vi "ADC Get Current Setup.vi"(8 "error in":errorcluster, 11 "adc session in":T14={"niScope"={"channel cfg"=[], "sessions"=[], "multi cards"=FALSE, "channels"=0, "type"=enum."n/a", "memory [B/chn]"=0, "ext. clock [Hz]"=0.0, "samples count"=0, "use streaming"=FALSE, "proc setup"={"packet size [smpl]"=0, "current timeout [s]"=0.0, "blk2blk timeout [s]"=0.0, "event time"=timestamp(0 s since 1904-01-01), "temp sampl T [s]"=0.0, "data queue"=refnum, "stop notifier"=refnum, "proc ref"=refnum}, "sample width [B]"=0, "ranges [V]"=[], "trigger setup"={"coupling"=1, "level [V]"=0.0, "slope"=0, "mode"=enum."Immediate", "pre-trigger [%]"=0.0}, "fs [Hz]"=0.0, "bitres [bit]"=0, "clock source"=enum."VAL_NO_SOURCE"}, "3458A"={"channels"=[], "sync unit"={"VISA"="", "type"=enum."Picotest U6200A"}, "awg unit"={"type"=enum."Agilent 331xxA to 332xxA", "VISA"="", "enable 10MHz ref"=FALSE, "cmi ckd2"={"VISA"="", "clock source"=enum."Auto", "manual ref clk"=FALSE, "ref clock [Hz]"=0.0, "div mode"=enum."Set divisor directly"}, "cmi sync v3"={"VISA"="", "baud rate [bd/s]"=115200, "source"=enum."Auto", "hv range"=enum."1kV", "fsrc is fixed"=FALSE, "fsrc [Hz]"=10000000.0, "freq integ [s]"=1.0, "freq filter"=5, "trig level"=enum."TTL 5V", "chn1 mode"=enum."Source divider", "chn1 level"=enum."Positive 5V", "chn2 mode"=enum."Source divider", "chn2 level"=enum."Positive 5V", "chn2 div"=1, "chn3 mode"=enum."Chn 1 Active", "chn3 level"=enum."Positive 5V", "chn1 div entry"=enum."Calculate nearest divisor from measured fx", "chn1 dev limit [%]"=1.0, "chn1 check dev"=FALSE}, "trigger"={"source"=enum."Immediate", "slope"=enum."POS", "coupling"=enum."DC", "level [V]"=0.0, "hysteresis [V]"=0.0, "pre-trigger [%]"=0.0}, "HMF2500 cfg"={"Baud Rate"=9600, "Parity"=0, "Data Bits"=8, "Flow Control"=4}}, "sync mode"=enum."MASTER-SLAVE, MASTER clocked by TIMER", "streaming mode"=FALSE, "idn mode"=enum."Auto", "sampling mode"=enum."DCV", "sample memory [B]"=0, "proc setup"={"channel id"=0, "packet size [smpl]"=0, "current timeout [s]"=0.0, "blk2blk timeout [s]"=0.0, "event time"=timestamp(0 s since 1904-01-01), "stop notifier"=refnum, "data queues"=[], "proc refs"=[], "bus semaphore"=refnum}, "sample size [B]"=0, "sample count"=0, "aux data"={"channel id"=0, "valid?"=[], "gain [V]"=[], "timestamp [s]"=[], "Ts [s]"=0.0, "abs timestamp"=timestamp(0 s since 1904-01-01), "t [deg C]"=[], "multiplex timestamp [s]"=-1.0, "only multiplex?"=FALSE, "multiplex smpl offset"=0, "overflow?"=FALSE}, "ranges [V]"=[], "aperture [s]"=0.0, "LEVEL trigger"={"edge"=enum."POS", "level [V]"=0.0, "coupling"=enum."DC"}, "trigger mode"=enum."AUTO", "measure temp.?"=FALSE, "disp mesages"=[], "shared bus?"=FALSE, "disable display?"=FALSE, "aper mode"=enum."Manual", "aper rules"=[], "multiplex"={"cycles"=0, "delay [s]"=0.0, "enabled"=FALSE, "overhead [s]"=1.0, "tot smpls"=0, "sub-rec"=0, "overhead [%]"=0.0, "emulated"=FALSE}, "F8588 lpf"=enum."Off", "F8588 pll"=enum."Off", "F8588 couple"=enum."DC, auto", "fs"={"freq mode"=enum."fs or Ts", "fs [Hz]"=0.0, "fref [Hz]"=0.0, "mul"=0.0, "div"=0.0}, "fs mode"=enum."fs or Ts"}, "dsdll"={"dsdll"={"dsdll path"=path "", "dsdll handle"=[], "output devices"=[], "capture devices"=[]}, "channels"=0, "device id"=0, "channel idns"=[], "proc setup"={"packet size [smpl]"=0, "current timeout [s]"=0.0, "blk2blk timeout [s]"=0.0, "event time"=timestamp(0 s since 1904-01-01), "data queue"=refnum, "stop notifier"=refnum, "proc ref"=refnum}, "samples count"=0, "fs [Hz]"=0.0}, "type"=enum."niScope", "channel idn str"=[], "aux instr idn str"=[], "modified?"=FALSE, "simadc"={"channels"=[], "range [V]"=0.0, "Ts step [s]"=0.0, "time [s]"=0.0, "fs [Hz]"=0.0, "count"=0, "smpl offset"=0, "set count"=0, "bit res"=0}, "force rst?"=FALSE, "exit mode"=enum."Immediate reset", "exit dly"=0.0, "exit tmr"=timestamp(0 s since 1904-01-01), "busy?"=FALSE, "accessed?"=FALSE, "multiplex"={"Type"=enum."Dummy", "gen com ssn"={"visa"="", "primary"=enum."None", "secondary"=enum."None", "channels"=[]}, "delay before [s]"=0.0, "delay post [s]"=0.0, "sequence"=[], "enabled"=FALSE, "ref timestamp [s]"=0.0, "idn string"="", "dev niScope"="", "niScope idx"=0, "QPMX ssn"={"visa"="", "switch mode"=enum."Switched by TWM", "sequence"=[], "timing delays"=[], "polarity"=enum."Positive", "ss delay (s)"=2.0, "internal timer (s)"=1.0, "Last loaded sequence file"=path "", "startup delay (s)"=2.0}, "VISA mux ssn"={"VISA"="", "paths"=[], "idn command"="", "serial cfg"={"Baud rate"=9600, "Data bits"=8, "Parity"=0, "Stop bits"=10, "Flow control"=0, "End Mode Read"=enum."None", "End Mode Write"=enum."None", "Term character"=0, "Term enable"=FALSE}}}, "keysight dso"={"VISA"="", "channels"=[], "bw limit [Hz]"=0.0, "resolution"=enum."Basic", "trig noise reject"=enum."Normal", "N"=0, "trigger config"={"trigger source"=enum."Immediate", "trigger slope"=enum."Negative", "level [V]"=0.0, "hysteresis [V]"=0.001, "pre-trig [%]"=50}, "fs [Hz]"=0.0, "timeout stop"=timestamp(0 s since 1904-01-01), "waiting for opc"=FALSE, "fetch offset [smpl]"=0, "abs timestamp"=timestamp(0 s since 1904-01-01), "ranges [V]"=[], "decimation"=1.0, "ext ref"=FALSE, "emulate aperture"=FALSE, "model"=enum."DSO91304"}, "cdaq"={"mclk [Hz]"=12800000.0, "ADC task"="", "mclk reference"="", "fs [Hz]"=50000.0, "queue adc cmd"=refnum, "queue adc data"=refnum, "adc proc ref"=refnum, "channels"=[], "last channels"=[], "timeout"=timestamp(0 s since 1904-01-01), "N"=1000, "mclk mode"=enum."Free running", "ext mclk source"=""}, "ignore overload"=FALSE, "ADS127L21"={"VISA"="", "chn list"=[], "record size"=0, "phys. channels"=0, "adc fifo size"=0, "channels"=[], "ext refclk?"=FALSE, "fs [Hz]"=0.0, "ext refclk [Hz]"=0.0, "meas refclk [Hz]"=0.0, "EXTOUT mode"=enum."ADCCLK", "EXTOUT polarity"=enum."NORM", "EXTOUT divisor"=0}} {"ADS127L21"."channels"."Channel" min=1 max=8 step=1; "cdaq"."last channels"."Channel id" min=0 step=1; "cdaq"."channels"."Channel id" min=0 step=1; "keysight dso"."decimation" min=1.0; "keysight dso"."bw limit [Hz]" format="%#_6p"; "keysight dso"."channels"."Offset [V]" format="%#_6p"; "keysight dso"."channels"."Range [Vpk]" min=0.0 format="%#_6p"; "keysight dso"."channels"."Channel" min=1; "multiplex"."VISA mux ssn"."serial cfg"."Flow control" items=["None", "XON/XOFF", "CTS/RTS", "XON/XOFF + CTS/RTS", "DTR/DSR", "XON/XOFF + DTR/DSR"]; "multiplex"."VISA mux ssn"."serial cfg"."Stop bits" items=["1 bit"=10, "1.5 bits"=15, "2 bits"=20]; "multiplex"."VISA mux ssn"."serial cfg"."Parity" items=["None", "Odd", "Even", "Mark", "Space"]; "multiplex"."VISA mux ssn"."serial cfg"."Data bits" items=["5 bits"=5, "6 bits"=6, "7 bits"=7, "8 bits"=8]; "multiplex"."VISA mux ssn"."serial cfg"."Baud rate" items=["150 Bd"=150, "300 Bd"=300, "600 Bd"=600, "1200 Bd"=1200, "2400 Bd"=2400, "4800 Bd"=4800, "9600 Bd"=9600, "19.2 kBd"=19200, "38.4 kBd"=38400, "57.6 kBd"=57600, "115.2 kBd"=115200]; "multiplex"."QPMX ssn"."startup delay (s)" min=0.0 step=1.0; "multiplex"."QPMX ssn"."internal timer (s)" min=0.0 step=1.0; "multiplex"."QPMX ssn"."ss delay (s)" min=0.0 step=1.0; "multiplex"."QPMX ssn"."timing delays" min=1 max=255 step=1; "3458A"."awg unit"."HMF2500 cfg"."Flow Control" items=["None", "XON/XOFF", "RTS/CTS", "XON/XOFF & RTS/CTS", "DTR/DSR", "XON/XOFF & DTR/DSR"]; "3458A"."awg unit"."HMF2500 cfg"."Data Bits" items=["7"=7, "8"=8]; "3458A"."awg unit"."HMF2500 cfg"."Parity" items=["None", "Odd", "Even", "Mark", "Space"]; "3458A"."awg unit"."HMF2500 cfg"."Baud Rate" items=["300"=300, "600"=600, "1200"=1200, "2400"=2400, "4800"=4800, "9600"=9600, "19200"=19200]; "3458A"."awg unit"."cmi sync v3"."chn2 div" min=1 max=100000000 step=1; "3458A"."awg unit"."cmi sync v3"."fsrc [Hz]" format="%_8p"; "3458A"."channels"."Range [Vpk]" min=0.0; "niScope"."trigger setup"."pre-trigger [%]" format="%.2f"; "niScope"."trigger setup"."level [V]" format="%.2f"; "niScope"."trigger setup"."coupling" items=["AC"=0, "DC"=1, "HF Reject"=3, "LF Reject"=4, "AC Plus HF Reject"=1001]; "niScope"."channel cfg"."Range [Vpk]" min=0.0; "niScope"."channel cfg"."Channel" min=0}) -> (0 "error out":errorcluster, 1 "device specific attributes":T11[](array[typedef]), 2 "common attributes":T6, 3 "adc session out":T14={"niScope"={"channel cfg"=[], "sessions"=[], "multi cards"=FALSE, "channels"=0, "type"=enum."n/a", "memory [B/chn]"=0, "ext. clock [Hz]"=0.0, "samples count"=0, "use streaming"=FALSE, "proc setup"={"packet size [smpl]"=0, "current timeout [s]"=0.0, "blk2blk timeout [s]"=0.0, "event time"=timestamp(0 s since 1904-01-01), "temp sampl T [s]"=0.0, "data queue"=refnum, "stop notifier"=refnum, "proc ref"=refnum}, "sample width [B]"=0, "ranges [V]"=[], "trigger setup"={"coupling"=1, "level [V]"=0.0, "slope"=0, "mode"=enum."Immediate", "pre-trigger [%]"=0.0}, "fs [Hz]"=0.0, "bitres [bit]"=0, "clock source"=enum."VAL_NO_SOURCE"}, "3458A"={"channels"=[], "sync unit"={"VISA"="", "type"=enum."Picotest U6200A"}, "awg unit"={"type"=enum."Agilent 331xxA to 332xxA", "VISA"="", "enable 10MHz ref"=FALSE, "cmi ckd2"={"VISA"="", "clock source"=enum."Auto", "manual ref clk"=FALSE, "ref clock [Hz]"=0.0, "div mode"=enum."Set divisor directly"}, "cmi sync v3"={"VISA"="", "baud rate [bd/s]"=115200, "source"=enum."Auto", "hv range"=enum."1kV", "fsrc is fixed"=FALSE, "fsrc [Hz]"=10000000.0, "freq integ [s]"=1.0, "freq filter"=5, "trig level"=enum."TTL 5V", "chn1 mode"=enum."Source divider", "chn1 level"=enum."Positive 5V", "chn2 mode"=enum."Source divider", "chn2 level"=enum."Positive 5V", "chn2 div"=1, "chn3 mode"=enum."Chn 1 Active", "chn3 level"=enum."Positive 5V", "chn1 div entry"=enum."Calculate nearest divisor from measured fx", "chn1 dev limit [%]"=1.0, "chn1 check dev"=FALSE}, "trigger"={"source"=enum."Immediate", "slope"=enum."POS", "coupling"=enum."DC", "level [V]"=0.0, "hysteresis [V]"=0.0, "pre-trigger [%]"=0.0}, "HMF2500 cfg"={"Baud Rate"=9600, "Parity"=0, "Data Bits"=8, "Flow Control"=4}}, "sync mode"=enum."MASTER-SLAVE, MASTER clocked by TIMER", "streaming mode"=FALSE, "idn mode"=enum."Auto", "sampling mode"=enum."DCV", "sample memory [B]"=0, "proc setup"={"channel id"=0, "packet size [smpl]"=0, "current timeout [s]"=0.0, "blk2blk timeout [s]"=0.0, "event time"=timestamp(0 s since 1904-01-01), "stop notifier"=refnum, "data queues"=[], "proc refs"=[], "bus semaphore"=refnum}, "sample size [B]"=0, "sample count"=0, "aux data"={"channel id"=0, "valid?"=[], "gain [V]"=[], "timestamp [s]"=[], "Ts [s]"=0.0, "abs timestamp"=timestamp(0 s since 1904-01-01), "t [deg C]"=[], "multiplex timestamp [s]"=-1.0, "only multiplex?"=FALSE, "multiplex smpl offset"=0, "overflow?"=FALSE}, "ranges [V]"=[], "aperture [s]"=0.0, "LEVEL trigger"={"edge"=enum."POS", "level [V]"=0.0, "coupling"=enum."DC"}, "trigger mode"=enum."AUTO", "measure temp.?"=FALSE, "disp mesages"=[], "shared bus?"=FALSE, "disable display?"=FALSE, "aper mode"=enum."Manual", "aper rules"=[], "multiplex"={"cycles"=0, "delay [s]"=0.0, "enabled"=FALSE, "overhead [s]"=1.0, "tot smpls"=0, "sub-rec"=0, "overhead [%]"=0.0, "emulated"=FALSE}, "F8588 lpf"=enum."Off", "F8588 pll"=enum."Off", "F8588 couple"=enum."DC, auto", "fs"={"freq mode"=enum."fs or Ts", "fs [Hz]"=0.0, "fref [Hz]"=0.0, "mul"=0.0, "div"=0.0}, "fs mode"=enum."fs or Ts"}, "dsdll"={"dsdll"={"dsdll path"=path "", "dsdll handle"=[], "output devices"=[], "capture devices"=[]}, "channels"=0, "device id"=0, "channel idns"=[], "proc setup"={"packet size [smpl]"=0, "current timeout [s]"=0.0, "blk2blk timeout [s]"=0.0, "event time"=timestamp(0 s since 1904-01-01), "data queue"=refnum, "stop notifier"=refnum, "proc ref"=refnum}, "samples count"=0, "fs [Hz]"=0.0}, "type"=enum."niScope", "channel idn str"=[], "aux instr idn str"=[], "modified?"=FALSE, "simadc"={"channels"=[], "range [V]"=0.0, "Ts step [s]"=0.0, "time [s]"=0.0, "fs [Hz]"=0.0, "count"=0, "smpl offset"=0, "set count"=0, "bit res"=0}, "force rst?"=FALSE, "exit mode"=enum."Immediate reset", "exit dly"=0.0, "exit tmr"=timestamp(0 s since 1904-01-01), "busy?"=FALSE, "accessed?"=FALSE, "multiplex"={"Type"=enum."Dummy", "gen com ssn"={"visa"="", "primary"=enum."None", "secondary"=enum."None", "channels"=[]}, "delay before [s]"=0.0, "delay post [s]"=0.0, "sequence"=[], "enabled"=FALSE, "ref timestamp [s]"=0.0, "idn string"="", "dev niScope"="", "niScope idx"=0, "QPMX ssn"={"visa"="", "switch mode"=enum."Switched by TWM", "sequence"=[], "timing delays"=[], "polarity"=enum."Positive", "ss delay (s)"=2.0, "internal timer (s)"=1.0, "Last loaded sequence file"=path "", "startup delay (s)"=2.0}, "VISA mux ssn"={"VISA"="", "paths"=[], "idn command"="", "serial cfg"={"Baud rate"=9600, "Data bits"=8, "Parity"=0, "Stop bits"=10, "Flow control"=0, "End Mode Read"=enum."None", "End Mode Write"=enum."None", "Term character"=0, "Term enable"=FALSE}}}, "keysight dso"={"VISA"="", "channels"=[], "bw limit [Hz]"=0.0, "resolution"=enum."Basic", "trig noise reject"=enum."Normal", "N"=0, "trigger config"={"trigger source"=enum."Immediate", "trigger slope"=enum."Negative", "level [V]"=0.0, "hysteresis [V]"=0.001, "pre-trig [%]"=50}, "fs [Hz]"=0.0, "timeout stop"=timestamp(0 s since 1904-01-01), "waiting for opc"=FALSE, "fetch offset [smpl]"=0, "abs timestamp"=timestamp(0 s since 1904-01-01), "ranges [V]"=[], "decimation"=1.0, "ext ref"=FALSE, "emulate aperture"=FALSE, "model"=enum."DSO91304"}, "cdaq"={"mclk [Hz]"=12800000.0, "ADC task"="", "mclk reference"="", "fs [Hz]"=50000.0, "queue adc cmd"=refnum, "queue adc data"=refnum, "adc proc ref"=refnum, "channels"=[], "last channels"=[], "timeout"=timestamp(0 s since 1904-01-01), "N"=1000, "mclk mode"=enum."Free running", "ext mclk source"=""}, "ignore overload"=FALSE, "ADS127L21"={"VISA"="", "chn list"=[], "record size"=0, "phys. channels"=0, "adc fifo size"=0, "channels"=[], "ext refclk?"=FALSE, "fs [Hz]"=0.0, "ext refclk [Hz]"=0.0, "meas refclk [Hz]"=0.0, "EXTOUT mode"=enum."ADCCLK", "EXTOUT polarity"=enum."NORM", "EXTOUT divisor"=0}} {"ADS127L21"."channels"."Channel" min=1 max=8 step=1; "cdaq"."last channels"."Channel id" min=0 step=1; "cdaq"."channels"."Channel id" min=0 step=1; "keysight dso"."decimation" min=1.0; "keysight dso"."bw limit [Hz]" format="%#_6p"; "keysight dso"."channels"."Offset [V]" format="%#_6p"; "keysight dso"."channels"."Range [Vpk]" min=0.0 format="%#_6p"; "keysight dso"."channels"."Channel" min=1; "multiplex"."VISA mux ssn"."serial cfg"."Flow control" items=["None", "XON/XOFF", "CTS/RTS", "XON/XOFF + CTS/RTS", "DTR/DSR", "XON/XOFF + DTR/DSR"]; "multiplex"."VISA mux ssn"."serial cfg"."Stop bits" items=["1 bit"=10, "1.5 bits"=15, "2 bits"=20]; "multiplex"."VISA mux ssn"."serial cfg"."Parity" items=["None", "Odd", "Even", "Mark", "Space"]; "multiplex"."VISA mux ssn"."serial cfg"."Data bits" items=["5 bits"=5, "6 bits"=6, "7 bits"=7, "8 bits"=8]; "multiplex"."VISA mux ssn"."serial cfg"."Baud rate" items=["150 Bd"=150, "300 Bd"=300, "600 Bd"=600, "1200 Bd"=1200, "2400 Bd"=2400, "4800 Bd"=4800, "9600 Bd"=9600, "19.2 kBd"=19200, "38.4 kBd"=38400, "57.6 kBd"=57600, "115.2 kBd"=115200]; "multiplex"."QPMX ssn"."startup delay (s)" min=0.0 step=1.0; "multiplex"."QPMX ssn"."internal timer (s)" min=0.0 step=1.0; "multiplex"."QPMX ssn"."ss delay (s)" min=0.0 step=1.0; "multiplex"."QPMX ssn"."timing delays" min=1 max=255 step=1; "3458A"."awg unit"."HMF2500 cfg"."Flow Control" items=["None", "XON/XOFF", "RTS/CTS", "XON/XOFF & RTS/CTS", "DTR/DSR", "XON/XOFF & DTR/DSR"]; "3458A"."awg unit"."HMF2500 cfg"."Data Bits" items=["7"=7, "8"=8]; "3458A"."awg unit"."HMF2500 cfg"."Parity" items=["None", "Odd", "Even", "Mark", "Space"]; "3458A"."awg unit"."HMF2500 cfg"."Baud Rate" items=["300"=300, "600"=600, "1200"=1200, "2400"=2400, "4800"=4800, "9600"=9600, "19200"=19200]; "3458A"."awg unit"."cmi sync v3"."chn2 div" min=1 max=100000000 step=1; "3458A"."awg unit"."cmi sync v3"."fsrc [Hz]" format="%_8p"; "3458A"."channels"."Range [Vpk]" min=0.0; "niScope"."trigger setup"."pre-trigger [%]" format="%.2f"; "niScope"."trigger setup"."level [V]" format="%.2f"; "niScope"."trigger setup"."coupling" items=["AC"=0, "DC"=1, "HF Reject"=3, "LF Reject"=4, "AC Plus HF Reject"=1001]; "niScope"."channel cfg"."Range [Vpk]" min=0.0; "niScope"."channel cfg"."Channel" min=0})   [LabVIEW 2020]
doc: "Returns current setup of the ADC (from session) so it will correctly work only after 'ADC Setup Virtual Channels'. It also returns device specific attributes as and array of names and text values."
uses:
  ADC Session.ctl
  drivers/niScope/niScope Session.ctl
  drivers/niScope/niScope Virtual Channel Config.ctl
  drivers/niScope/niScope Virtual Channel Mode.ctl
  drivers/niScope/niScope Virtual Channel Input Z.ctl
  drivers/niScope/niScope Virtual Channel Coupling.ctl
  drivers/niScope/niScope Type.ctl
  drivers/niScope/niScope Digitizing Process Options.ctl
  drivers/niScope/niScope Data Packet.ctl
  drivers/niScope/niScope Trigger Setup.ctl
  <instrlib>/niScope/Controls/niScope trigger coupling.ctl
  <instrlib>/niScope/Controls/niScope trigger slope.ctl
  drivers/niScope/niScope Reference Clock.ctl
  drivers/DMM/3458A Digitizer Session.ctl
  drivers/DMM/3458A Virtual Channel Config.ctl
  drivers/Counter/Counter Session.ctl
  drivers/Counter/Counter Type.ctl
  drivers/AWG/AWG Session.ctl
  drivers/AWG/AWG Type.ctl
  drivers/AWG/CMI Clock Divider v2/CMI ckd2 Session.ctl
  drivers/AWG/CMI Clock Divider v2/CMI ckd2 Source Mode.ctl
  drivers/AWG/CMI Clock Divider v2/CMI ckd2 Divisor Mode.ctl
  drivers/AWG/CMI Sync V3/CMI Sync V3 session.ctl
  drivers/AWG/CMI Sync V3/Configure/CMI Sync V3 Reference Clock Source.ctl
  drivers/AWG/CMI Sync V3/Configure/CMI Sync V3 HV input Range.ctl
  drivers/AWG/CMI Sync V3/Configure/CMI Sync V3 Trigger Input Level.ctl
  drivers/AWG/CMI Sync V3/Configure/CMI Sync V3 Channel 1 Mode.ctl
  drivers/AWG/CMI Sync V3/Configure/CMI Sync V3 Channel Output Levels.ctl
  drivers/AWG/CMI Sync V3/Configure/CMI Sync V3 Channel 2 Mode.ctl
  drivers/AWG/CMI Sync V3/Configure/CMI Sync V3 Channel 3 Mode.ctl
  drivers/AWG/CMI Sync V3/Configure/CMI Sync V3 Channel 1 Divisor Entry Mode.ctl
  ADC Trig Config.ctl
  ADC Trig Mode Source.ctl
  ADC Trig Slope.ctl
  ADC Trig Coupling.ctl
  drivers/AWG/RaS HMF2500/HMF2500 Config.ctl
  drivers/DMM/3458A Sync Mode.ctl
  drivers/DMM/3458A Idn Mode.ctl
  drivers/DMM/3458A Digitizing Low Levels/Configure/Sampling Mode.ctl
  drivers/DMM/3458A Digitizing Process Options.ctl
  drivers/DMM/3458A Data Packet.ctl
  drivers/DMM/3458A Aux Record Data.ctl
  drivers/DMM/3458A Digitizing Low Levels/Configure/Level Setup.ctl
  drivers/DMM/3458A Digitizing Low Levels/Configure/First Sample Trigger.ctl
  drivers/DMM/3458A Aperture Selection Mode.ctl
  drivers/DMM/3458A Multiplexing Config.ctl
  drivers/Fluke 8588A/F8588A Low Pass Filter.ctl
  drivers/Fluke 8588A/F8588A Phase Lock.ctl
  drivers/Fluke 8588A/F8588A Coupling.ctl
  drivers/DMM/3458A Sampling Rate.ctl
  drivers/AWG/AWG Clock Setup Mode.ctl
  drivers/DMM/3458A Sample Rate Mode.ctl
  drivers/dsdll/DSDLL Session.ctl
  drivers/dsdll/dsdll/dsdll_instance.ctl
  drivers/dsdll/dsdll/dsdll_device_record.ctl
  drivers/dsdll/DSDLL Process Config.ctl
  drivers/dsdll/DSDLL Data Packet.ctl
  ADC Type.ctl
  drivers/simulated_adc/SimAdc Config.ctl
  drivers/simulated_adc/SimAdc Channel Cfg.ctl
  ADC On Close Action.ctl
  Multiplexer/MPX Session.ctl
  Multiplexer/MPX Type.ctl
  drivers/Multiplexers/Generic COM/GCOMM Session.ctl
  drivers/Multiplexers/Generic COM/GCOMM Signal.ctl
  drivers/Multiplexers/Generic COM/GCOMM Virtual Channel.ctl
  drivers/Multiplexers/Generic COM/GCOMM Logic State.ctl
  drivers/Multiplexers/Generic COM/QPMX Session.ctl
  drivers/Multiplexers/QPMX/QPMX switch mode.ctl
  drivers/Multiplexers/QPMX/QPMX polarity.ctl
  drivers/Multiplexers/Generic VISA commands/GVISA Mux Session.ctl
  drivers/Multiplexers/Generic VISA commands/GVISA Mux Path Entry.ctl
  drivers/Multiplexers/Generic VISA commands/met_serial_setup.ctl
  drivers/Agilent DSO 90000/Virtual Digitizer/KeDSO session.ctl
  drivers/Agilent DSO 90000/Virtual Digitizer/KeDSO Virtual Channel.ctl
  drivers/Agilent DSO 90000/Virtual Digitizer/KeDSO High Resolution Mode.ctl
  drivers/Agilent DSO 90000/Virtual Digitizer/KeDSO Trigger Setup.ctl
  drivers/Agilent DSO 90000/Virtual Digitizer/KeDSO Trigger Source.ctl
  drivers/Agilent DSO 90000/Public/Utility/DSO type.ctl
  drivers/cdaq/cDAQ Session.ctl
  drivers/cdaq/low_level_old/cdaq_anal_adc_command.ctl
  drivers/cdaq/low_level_old/cdaq_anal_adc_data.ctl
  drivers/cdaq/cDAQ Virtual Channel.ctl
  drivers/cdaq/cDAQ Master Clock Mode.ctl
  drivers/CMI_ADS127L21/CMI ADS127L21 - Session.ctl
  drivers/CMI_ADS127L21/CMI ADS127L21 - Record Channel.ctl
  drivers/CMI_ADS127L21/CMI ADS127L21 - Input Range.ctl
  drivers/CMI_ADS127L21/CMI ADS127L21 - Input Mode.ctl
  drivers/CMI_ADS127L21/CMI ADS127L21 - Input Impedance.ctl
  drivers/CMI_ADS127L21/CMI ADS127L21 - EXTOUT Mode.ctl
  drivers/CMI_ADS127L21/CMI ADS127L21 - EXTOUT Polarity.ctl
  ADC Attribute.ctl
  ADC Current Configuration.ctl
  drivers/DMM/3458A Virtual Digitizer.lvlib
  drivers/niScope/niScope Virtual Digitizer.lvlib
  drivers/Counter/Counter.lvlib
  drivers/AWG/AWG.lvlib
  drivers/DMM/3458A Digitizing Low Levels/3458A Digitizing Low Levels.lvlib
  drivers/dsdll/DSDLL Virtual Digitizer.lvlib
  drivers/dsdll/dsdll/dsdll.lvlib
  drivers/AWG/CMI Sync V3/CMI Sync Unit V3.lvlib
  drivers/Agilent DSO 90000/Agilent 90000 Series.lvlib
panel:
  in  "ads127 Impedance":T1
  in  "ads127 Mode":T2
  in  "Coupling 2":enum16{"DC", "DC50", "AC", "LFR1"}(ring)
  in  "Coupling":T3=enum."DC"
  in  "Input Z":T4
  in  "Mode":T5
  in  "3458A.sync mode":T12
  in  "3458A.sampling mode":T13
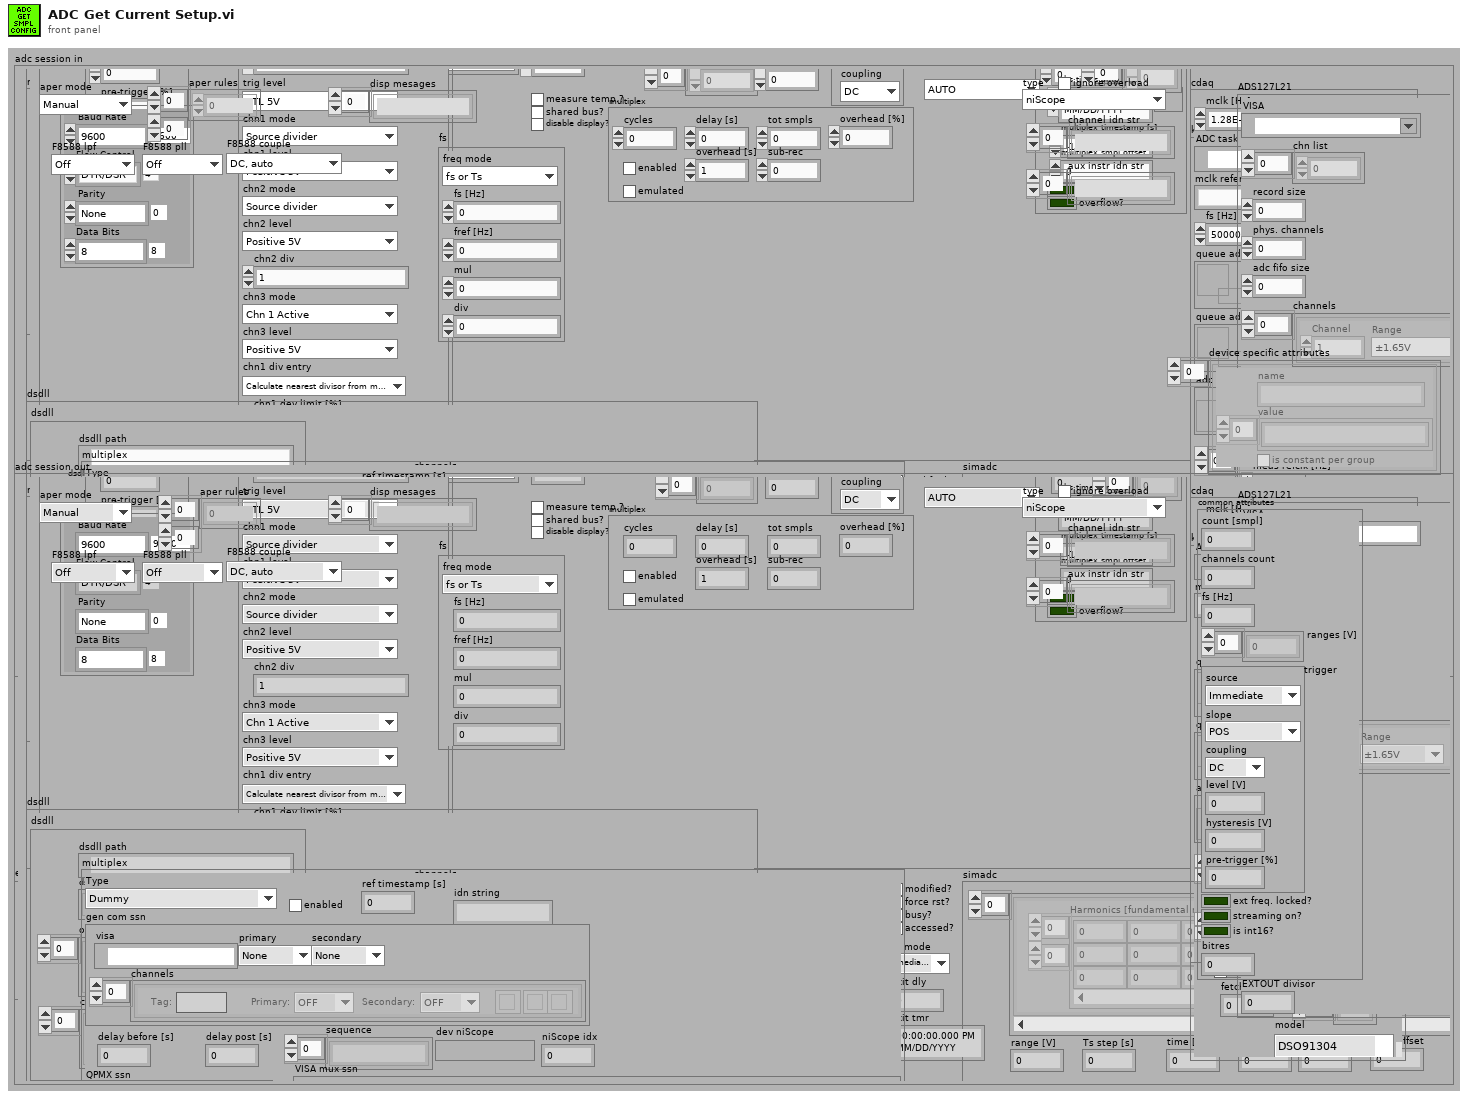
[diagram p1: front panel]
types:
  T1 = typedef "CMI ADS127L21 - Input Impedance.ctl" = enum16{"1M", "1k5"}
  T2 = typedef "CMI ADS127L21 - Input Mode.ctl" = enum16{"Normal", "Inverted", "GND"}
  T3 = typedef "niScope Virtual Digitizer.lvlib/niScope Virtual Channel Coupling.ctl" = enum16{"AC", "DC", "GND"}
  T4 = typedef "niScope Virtual Digitizer.lvlib/niScope Virtual Channel Input Z.ctl" = enum16{"1 MOhm", "50 Ohm"}
  T5 = typedef "niScope Virtual Digitizer.lvlib/niScope Virtual Channel Mode.ctl" = enum16{"Single ended", "Unbal. differential", "Differential"}
  T6 = typedef "ADC Current Configuration.ctl" = cluster{"count [smpl]":i64, "channels count":i32, "fs [Hz]":dbl, "ranges [V]":dbl[], "trigger":T7, "ext freq. locked?":bool, "streaming on?":bool, "is int16?":bool, "bitres":i32}
  T7 = typedef "ADC Trig Config.ctl" = cluster{"source":T8, "slope":T9, "coupling":T10, "level [V]":dbl, "hysteresis [V]":dbl, "pre-trigger [%]":dbl}
  T8 = typedef "ADC Trig Mode Source.ctl" = enum16{"Immediate", "External", "Level"}
  T9 = typedef "ADC Trig Slope.ctl" = enum16{"POS", "NEG"}
  T10 = typedef "ADC Trig Coupling.ctl" = enum16{"DC", "AC"}
  T11 = typedef "ADC Attribute.ctl" = cluster{"name":string, "value":string[], "is constant per group":bool}
  T12 = typedef "3458A Virtual Digitizer.lvlib/3458A Sync Mode.ctl" = enum16{"MASTER-SLAVE, MASTER clocked by TIMER", "MASTER-SLAVE, MASTER clocked by AWG", "ALL clocked by AWG", "MASTER-SLAVE, ALL clocked by TIMER", "ALL clocked by AWG with DFLL"}
  T13 = typedef "3458A Virtual Digitizer.lvlib/3458A Digitizing Low Levels.lvlib/Sampling Mode.ctl" = enum16{"DCV", "DSDC", "DSAC"}
  T14 = typedef "ADC Session.ctl" = cluster{"niScope":T15, "3458A":T23, "dsdll":T56, "type":T60, "channel idn str":string[], "aux instr idn str":string[], "modified?":bool, "simadc":T61, "force rst?":bool, "exit mode":T63, "exit dly":dbl, "exit tmr":timestamp, "busy?":bool, "accessed?":bool, "multiplex":T64, "keysight dso":T76, "cdaq":T82, "ignore overload":bool, "ADS127L21":T85}
  T15 = typedef "niScope Virtual Digitizer.lvlib/niScope Session.ctl" = cluster{"channel cfg":T16[], "sessions":refnum<k20>[], "multi cards":bool, "channels":i32, "type":T17, "memory [B/chn]":i32, "ext. clock [Hz]":dbl, "samples count":i64, "use streaming":bool, "proc setup":T18, "sample width [B]":i32, "ranges [V]":dbl[], "trigger setup":T19, "fs [Hz]":dbl, "bitres [bit]":i32, "clock source":T22}
  T16 = typedef "niScope Virtual Digitizer.lvlib/niScope Virtual Channel Config.ctl" = cluster{"Address":refnum<k15>, "Channel":i32, "Mode":T5, "Input Z":T4, "Coupling":T3, "Range [Vpk]":dbl, "btn clr":bool, "btn up":bool, "btn down":bool}
  T17 = typedef "niScope Virtual Digitizer.lvlib/niScope Type.ctl" = enum16{"n/a", "5922"}
  T18 = typedef "niScope Virtual Digitizer.lvlib/niScope Digitizing Process Options.ctl" = cluster{"packet size [smpl]":i64, "current timeout [s]":dbl, "blk2blk timeout [s]":dbl, "event time":timestamp, "temp sampl T [s]":dbl, "data queue":refnum<queue>, "stop notifier":refnum<notifier>, "proc ref":refnum<vi>}
  T19 = typedef "niScope Virtual Digitizer.lvlib/niScope Trigger Setup.ctl" = cluster{"coupling":T20, "level [V]":dbl, "slope":T21, "mode":enum16{"Immediate", "External", "Level"}, "pre-trigger [%]":dbl}
  T20 = typedef "niScope trigger coupling.ctl" = u16
  T21 = typedef "niScope trigger slope.ctl" = i32
  T22 = typedef "niScope Virtual Digitizer.lvlib/niScope Reference Clock.ctl" = enum16{"VAL_NO_SOURCE", "VAL_CLK_IN", "VAL_PXI_CLOCK", "VAL_EXTERNAL"}
  T23 = typedef "3458A Virtual Digitizer.lvlib/3458A Digitizer Session.ctl" = cluster{"channels":T24[], "sync unit":T25, "awg unit":T27, "sync mode":T12, "streaming mode":bool, "idn mode":T42, "sampling mode":T13, "sample memory [B]":i32, "proc setup":T43, "sample size [B]":i32, "sample count":i32, "aux data":T45, "ranges [V]":dbl[], "aperture [s]":dbl, "LEVEL trigger":T46, "trigger mode":T47, "measure temp.?":bool, "disp mesages":string[], "shared bus?":bool, "disable display?":bool, "aper mode":T48, "aper rules":dbl[][], "multiplex":T49, "F8588 lpf":T50, "F8588 pll":T51, "F8588 couple":T52, "fs":T53, "fs mode":T55}
  T24 = typedef "3458A Virtual Digitizer.lvlib/3458A Virtual Channel Config.ctl" = cluster{"VISA":refnum<visa-resource-name>, "Range [Vpk]":dbl, "btn clr":bool, "btn up":bool, "btn down":bool, "F8588":bool, "F8588 guard":bool}
  T25 = typedef "Counter.lvlib/Counter Session.ctl" = cluster{"VISA":refnum<visa-resource-name>, "type":T26}
  T26 = typedef "Counter.lvlib/Counter Type.ctl" = enum16{"Picotest U6200A", "dummy"}
  T27 = typedef "AWG.lvlib/AWG Session.ctl" = cluster{"type":T28, "VISA":refnum<visa-resource-name>, "enable 10MHz ref":bool, "cmi ckd2":T29, "cmi sync v3":T32, "trigger":T7, "HMF2500 cfg":T41}
  T28 = typedef "AWG.lvlib/AWG Type.ctl" = enum16{"Agilent 331xxA to 332xxA", "Agilent 335xxA to 336xxA", "Tektronix AFG3101C", "R&S HMF25xx", "CMI Clock Divider v2", "CMI Sync Unit V3", "dummy"}
  T29 = typedef "AWG.lvlib/CMI ckd2 Session.ctl" = cluster{"VISA":refnum<visa-resource-name>, "clock source":T30, "manual ref clk":bool, "ref clock [Hz]":dbl, "div mode":T31}
  T30 = typedef "AWG.lvlib/CMI ckd2 Source Mode.ctl" = enum16{"Auto", "LF clock", "HF clock", "Internal"}
  T31 = typedef "AWG.lvlib/CMI ckd2 Divisor Mode.ctl" = enum16{"Set divisor directly", "Set divisor by frequency"}
  T32 = typedef "AWG.lvlib/CMI Sync Unit V3.lvlib/CMI Sync V3 session.ctl" = cluster{"VISA":refnum<visa-resource-name>, "baud rate [bd/s]":i32, "source":T33, "hv range":T34, "fsrc is fixed":bool, "fsrc [Hz]":dbl, "freq integ [s]":dbl, "freq filter":i32, "trig level":T35, "chn1 mode":T36, "chn1 level":T37, "chn2 mode":T38, "chn2 level":T37, "chn2 div":i32, "chn3 mode":T39, "chn3 level":T37, "chn1 div entry":T40, "chn1 dev limit [%]":dbl, "chn1 check dev":bool}
  T33 = typedef "AWG.lvlib/CMI Sync Unit V3.lvlib/CMI Sync V3 Reference Clock Source.ctl" = enum16{"Auto", "Internal", "Logic", "Sine", "HV"}
  T34 = typedef "AWG.lvlib/CMI Sync Unit V3.lvlib/CMI Sync V3 HV input Range.ctl" = enum16{"10V", "60V", "250V", "1kV"}
  T35 = typedef "AWG.lvlib/CMI Sync Unit V3.lvlib/CMI Sync V3 Trigger Input Level.ctl" = enum16{"LVCMOS 3V3", "TTL 5V"}
  T36 = typedef "AWG.lvlib/CMI Sync Unit V3.lvlib/CMI Sync V3 Channel 1 Mode.ctl" = enum16{"Source divider", "DDS absolute", "DDS ratio", "DDS ratio M/N"}
  T37 = typedef "AWG.lvlib/CMI Sync Unit V3.lvlib/CMI Sync V3 Channel Output Levels.ctl" = enum16{"Positive 3V3", "Negative 3V3", "Positive 5V", "Negative 5V"}
  T38 = typedef "AWG.lvlib/CMI Sync Unit V3.lvlib/CMI Sync V3 Channel 2 Mode.ctl" = enum16{"Source divider", "Chn 1 divide"}
  T39 = typedef "AWG.lvlib/CMI Sync Unit V3.lvlib/CMI Sync V3 Channel 3 Mode.ctl" = enum16{"Chn 1 Active", "Chn 2 Active", "Chn 1 Trigger", "Chn 2 Trigger", "Gate", "PPS", "10MHz"}
  T40 = typedef "AWG.lvlib/CMI Sync Unit V3.lvlib/CMI Sync V3 Channel 1 Divisor Entry Mode.ctl" = enum16{"Set divisor directly", "Calculate nearest divisor from measured fx"}
  T41 = typedef "AWG.lvlib/HMF2500 Config.ctl" = cluster{"Baud Rate":u32, "Parity":u16, "Data Bits":u16, "Flow Control":u16}
  T42 = typedef "3458A Virtual Digitizer.lvlib/3458A Idn Mode.ctl" = enum16{"Auto", "Sequential (chn A, chn B, ...)", "From calibration string"}
  T43 = typedef "3458A Virtual Digitizer.lvlib/3458A Digitizing Process Options.ctl" = cluster{"channel id":i32, "packet size [smpl]":i32, "current timeout [s]":dbl, "blk2blk timeout [s]":dbl, "event time":timestamp, "stop notifier":refnum<notifier>, "data queues":refnum<queue>[], "proc refs":refnum<vi>[], "bus semaphore":T44}
  T44 = typedef "Semaphore RefNum" = refnum<k1>
  T45 = typedef "3458A Virtual Digitizer.lvlib/3458A Aux Record Data.ctl" = cluster{"channel id":i32, "valid?":bool[], "gain [V]":dbl[], "timestamp [s]":dbl[], "Ts [s]":dbl, "abs timestamp":timestamp, "t [deg C]":dbl[], "multiplex timestamp [s]":dbl, "only multiplex?":bool, "multiplex smpl offset":i64, "overflow?":bool}
  T46 = typedef "3458A Virtual Digitizer.lvlib/3458A Digitizing Low Levels.lvlib/Level Setup.ctl" = cluster{"edge":enum16{"POS", "NEG"}, "level [V]":dbl, "coupling":enum16{"DC", "AC"}}
  T47 = typedef "3458A Virtual Digitizer.lvlib/3458A Digitizing Low Levels.lvlib/First Sample Trigger.ctl" = enum16{"AUTO", "EXT", "SYN", "SGL", "HOLD", "LEVEL"}
  T48 = typedef "3458A Virtual Digitizer.lvlib/3458A Aperture Selection Mode.ctl" = enum16{"Manual", "Maximum", "Table"}
  T49 = typedef "3458A Virtual Digitizer.lvlib/3458A Multiplexing Config.ctl" = cluster{"cycles":i32, "delay [s]":dbl, "enabled":bool, "overhead [s]":dbl, "tot smpls":i64, "sub-rec":i32, "overhead [%]":dbl, "emulated":bool}
  T50 = typedef "F8588A Low Pass Filter.ctl" = enum16{"Off", "100 kHz", "3 MHz"}
  T51 = typedef "F8588A Phase Lock.ctl" = enum16{"Off", "1 MHz", "10 MHz"}
  T52 = typedef "F8588A Coupling.ctl" = enum16{"AC, 1 MOhm", "AC, 10 MOhm", "DC, 1 MOhm", "DC, 10 MOhm", "DC, auto"}
  T53 = typedef "3458A Virtual Digitizer.lvlib/3458A Sampling Rate.ctl" = cluster{"freq mode":T54, "fs [Hz]":dbl, "fref [Hz]":dbl, "mul":dbl, "div":dbl}
  T54 = typedef "AWG.lvlib/AWG Clock Setup Mode.ctl" = enum16{"fs or Ts", "fs or Ts with fref", "fref/N", "fref*M/N", "fref*Ratio"}
  T55 = typedef "3458A Sample Rate Mode.ctl" = enum16{"fs or Ts", "fs*M/N"}
  T56 = typedef "DSDLL Virtual Digitizer.lvlib/DSDLL Session.ctl" = cluster{"dsdll":T57, "channels":i32, "device id":i32, "channel idns":string[], "proc setup":T59, "samples count":i32, "fs [Hz]":dbl}
  T57 = typedef "dsdll.lvlib/dsdll_instance.ctl" = cluster{"dsdll path":path, "dsdll handle":u8[], "output devices":T58[], "capture devices":T58[]}
  T58 = typedef "dsdll.lvlib/dsdll_device_record.ctl" = cluster{"guid":u8[], "name":string}
  T59 = typedef "DSDLL Virtual Digitizer.lvlib/DSDLL Process Config.ctl" = cluster{"packet size [smpl]":i32, "current timeout [s]":dbl, "blk2blk timeout [s]":dbl, "event time":timestamp, "data queue":refnum<queue>, "stop notifier":refnum<notifier>, "proc ref":refnum<vi>}
  T60 = typedef "ADC Type.ctl" = enum16{"niScope", "3458A", "DirectSound DLL", "Keysight DSO", "cDAQ ADC", "CMI ADS127L21", "dummy"}
  T61 = typedef "SimAdc Config.ctl" = cluster{"channels":T62[], "range [V]":dbl, "Ts step [s]":dbl, "time [s]":dbl, "fs [Hz]":dbl, "count":i64, "smpl offset":i64, "set count":i64, "bit res":i32}
  T62 = typedef "SimAdc Channel Cfg.ctl" = cluster{"harmonics":dbl[][], "btn clear":bool, "noise":dbl, "fundamental [Hz]":dbl}
  T63 = typedef "ADC On Close Action.ctl" = enum16{"Immediate reset", "Delayed reset"}
  T64 = typedef "MPX Session.ctl" = cluster{"Type":T65, "gen com ssn":T66, "delay before [s]":dbl, "delay post [s]":dbl, "sequence":string[], "enabled":bool, "ref timestamp [s]":dbl, "idn string":string, "dev niScope":refnum<k15>, "niScope idx":i32, "QPMX ssn":T70, "VISA mux ssn":T73}
  T65 = typedef "MPX Type.ctl" = enum16{"Dummy", "Generic - COM port", "Generic - niScope PFI", "Generic - VISA commands", "QPMX"}
  T66 = typedef "GCOMM Session.ctl" = cluster{"visa":refnum<visa-resource-name>, "primary":T67, "secondary":T67, "channels":T68[]}
  T67 = typedef "GCOMM Signal.ctl" = enum16{"None", "DTR", "RTS"}
  T68 = typedef "GCOMM Virtual Channel.ctl" = cluster{"Primary:":T69, "Secondary:":T69, "btn clr":bool, "btn up":bool, "btn down":bool, "Tag:":string}
  T69 = typedef "GCOMM Logic State.ctl" = enum16{"OFF", "ON"}
  T70 = typedef "QPMX Session.ctl" = cluster{"visa":refnum<visa-resource-name>, "switch mode":T71, "sequence":bool[][], "timing delays":u32[], "polarity":T72, "ss delay (s)":dbl, "internal timer (s)":dbl, "Last loaded sequence file":path, "startup delay (s)":dbl}
  T71 = typedef "QPMX switch mode.ctl" = enum16{"Switched by TWM", "Switched by external clock", "Switched by internal clock"}
  T72 = typedef "QPMX polarity.ctl" = enum16{"Positive", "Negative"}
  T73 = typedef "GVISA Mux Session.ctl" = cluster{"VISA":refnum<visa-resource-name>, "paths":T74[], "idn command":string, "serial cfg":T75}
  T74 = typedef "GVISA Mux Path Entry.ctl" = cluster{"Tag:":string, "Command:":string, "btn clr":bool, "btn up":bool, "btn down":bool}
  T75 = typedef "met_serial_setup.ctl" = cluster{"Baud rate":i32, "Data bits":i32, "Parity":i32, "Stop bits":i32, "Flow control":i32, "End Mode Read":enum16{"None", "Last Bit", "TermChar"}, "End Mode Write":enum16{"None", "Last Bit", "TermChar"}, "Term character":u8, "Term enable":bool}
  T76 = typedef "KeDSO session.ctl" = cluster{"VISA":refnum<visa-resource-name>, "channels":T77[], "bw limit [Hz]":dbl, "resolution":T78, "trig noise reject":enum16{"Normal", "High Sensitivity"}, "N":i64, "trigger config":T79, "fs [Hz]":dbl, "timeout stop":timestamp, "waiting for opc":bool, "fetch offset [smpl]":i64, "abs timestamp":timestamp, "ranges [V]":dbl[], "decimation":dbl, "ext ref":bool, "emulate aperture":bool, "model":T81}
  T77 = typedef "KeDSO Virtual Channel.ctl" = cluster{"Channel":i32, "Range [Vpk]":dbl, "btn clr":bool, "btn up":bool, "btn down":bool, "Offset [V]":dbl, "Coupling":enum16{"DC", "DC50", "AC", "LFR1"}, "bw limit enab":bool}
  T78 = typedef "KeDSO High Resolution Mode.ctl" = enum16{"Basic", "High-res AUTO", "Min. 9-bits", "Min. 10-bits", "Min. 11-bits", "Min. 12-bits", "Fixed 11-bits", "Fixed 12-bits", "Fixed 13-bits", "Fixed 14-bits", "Fixed 15-bits", "Fixed 16-bits"}
  T79 = typedef "KeDSO Trigger Setup.ctl" = cluster{"trigger source":T80, "trigger slope":enum16{"Negative", "Positive", "Either"}, "level [V]":dbl, "hysteresis [V]":dbl, "pre-trig [%]":i32}
  T80 = typedef "KeDSO Trigger Source.ctl" = enum16{"Immediate", "Level", "AUX"}
  T81 = typedef "Agilent 90000 Series.lvlib/DSO type.ctl" = enum16{"DSO91304", "DSO91204", "DSO90804", "DSO90604", "DSO90404", "DSO90254", "DSA91304", "DSA91204", "DSA90804", "DSA90604", "DSA90404", "DSA90254", "DSO9104", "DSO9254", "DSO9404", "MSO9104", "MSO9254", "MSO9404", "MSO9064", "DSO9064", "DSOX91604", "DSOX92004", "DSOX92504", "DSOX92804", "DSOX93204", "DSO93004", "DSO9024H", "DSO9054H", "DSO9104H", "DSO9204H", "DSOS054A", "DSOS104A", "DSOS204A", "DSOS254A", "DSOS404A", "DSOS604A", "DSOS804A", "MSOS054A", "MSOS104A", "MSOS204A", "MSOS254A", "MSOS404A", "MSOS604A", "MSOS804A", "DSAX96204Q", "DSOX96204Q", "DSAX95004Q", "DSOX95004Q", "DSAX93304Q", "DSOX93304Q", "DSAX92504Q", "DSOX92504Q", "DSAX92004Q", "DSOX92004Q"}
  T82 = typedef "cDAQ Session.ctl" = cluster{"mclk [Hz]":dbl, "ADC task":refnum<k21>, "mclk reference":string, "fs [Hz]":dbl, "queue adc cmd":refnum<queue>, "queue adc data":refnum<queue>, "adc proc ref":refnum<vi>, "channels":T83[], "last channels":T83[], "timeout":timestamp, "N":i32, "mclk mode":T84, "ext mclk source":tag}
  T83 = typedef "cDAQ Virtual Channel.ctl" = cluster{"Device":tag, "Channel id":i32, "btn clr":bool, "btn up":bool, "btn down":bool}
  T84 = typedef "cDAQ Master Clock Mode.ctl" = enum16{"Free running", "Export master clock", "Import master clock"}
  T85 = typedef "CMI ADS127L21 - Session.ctl" = cluster{"VISA":refnum<visa-resource-name>, "chn list":i32[], "record size":i32, "phys. channels":i32, "adc fifo size":i32, "channels":T86[], "ext refclk?":bool, "fs [Hz]":dbl, "ext refclk [Hz]":dbl, "meas refclk [Hz]":dbl, "EXTOUT mode":T88, "EXTOUT polarity":T89, "EXTOUT divisor":i32}
  T86 = typedef "CMI ADS127L21 - Record Channel.ctl" = cluster{"Range":T87, "Channel":i32, "Mode":T2, "Impedance":T1}
  T87 = typedef "CMI ADS127L21 - Input Range.ctl" = enum16{"±1.65V", "±2V"}
  T88 = typedef "CMI ADS127L21 - EXTOUT Mode.ctl" = enum16{"ADCCLK", "REFCLK", "SMPLCLK", "FIRST"}
  T89 = typedef "CMI ADS127L21 - EXTOUT Polarity.ctl" = enum16{"NORM", "INV"}
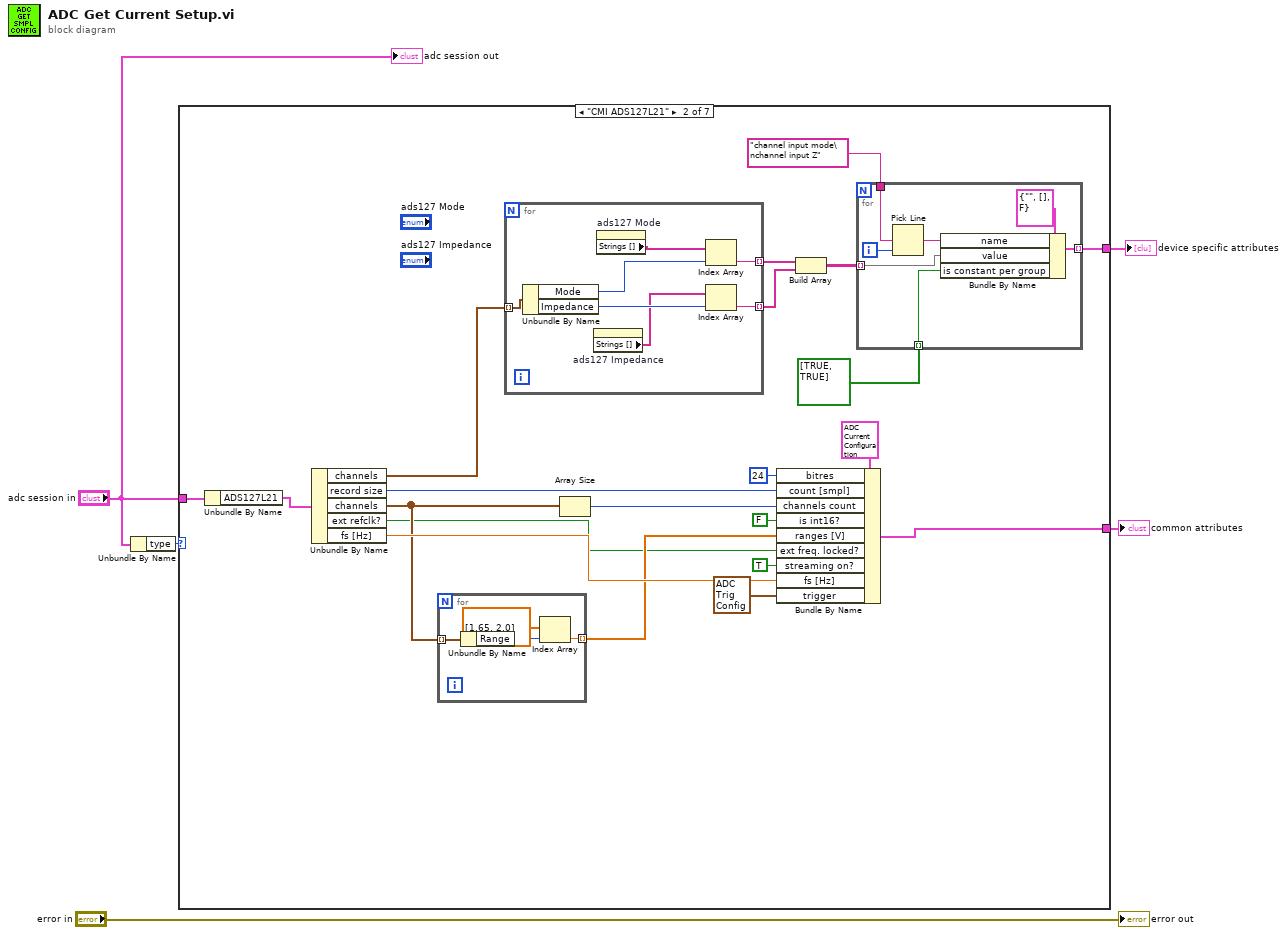
[diagram p0: block diagram]
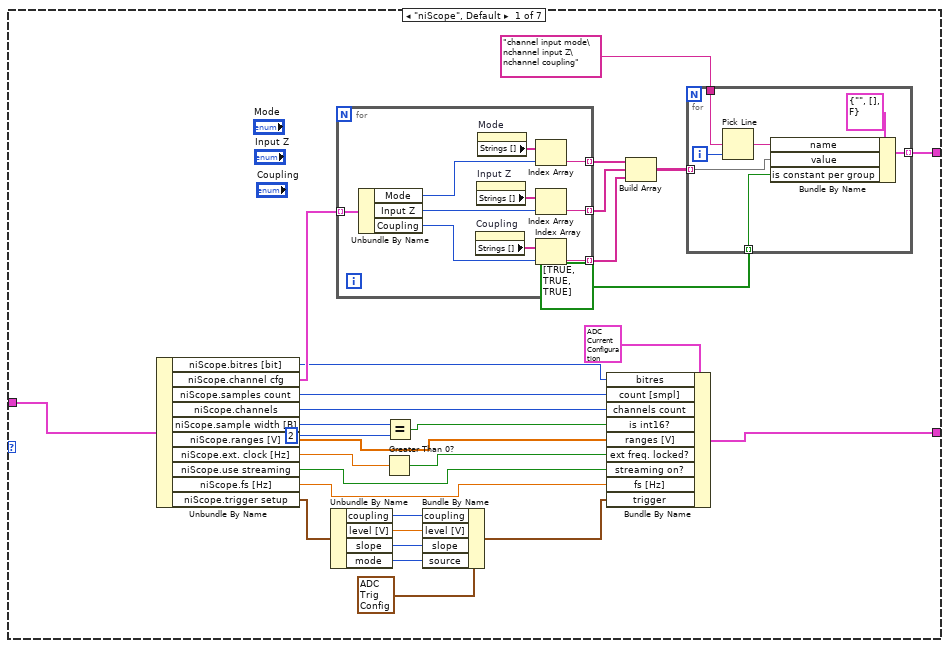
[diagram p2: hidden frame]
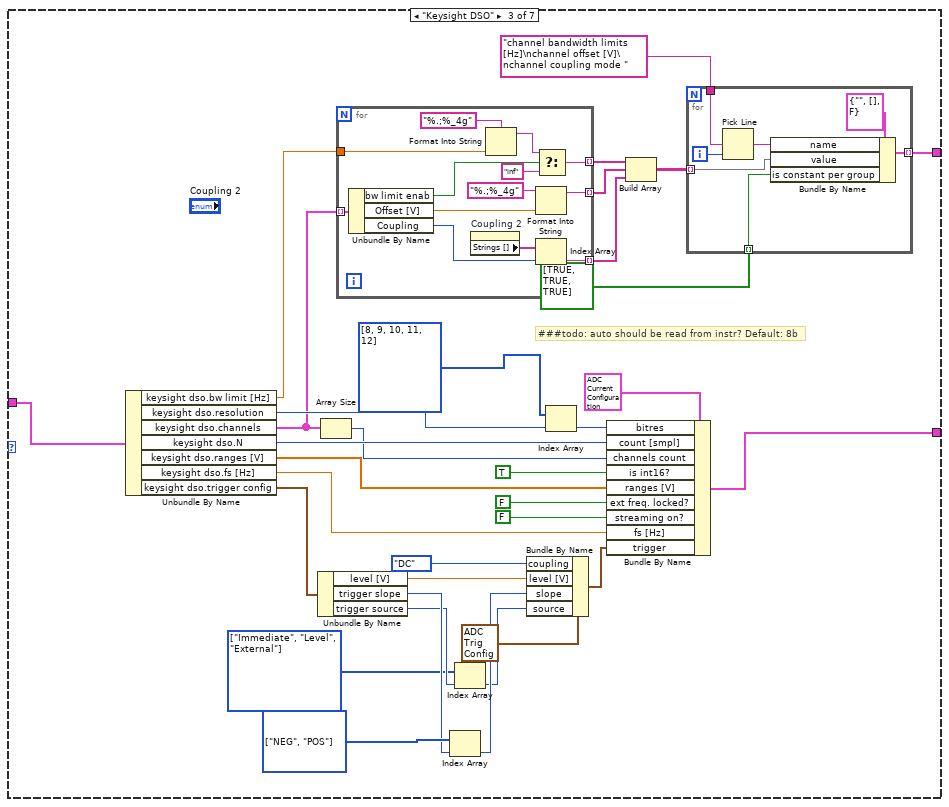
[diagram p3: hidden frame]
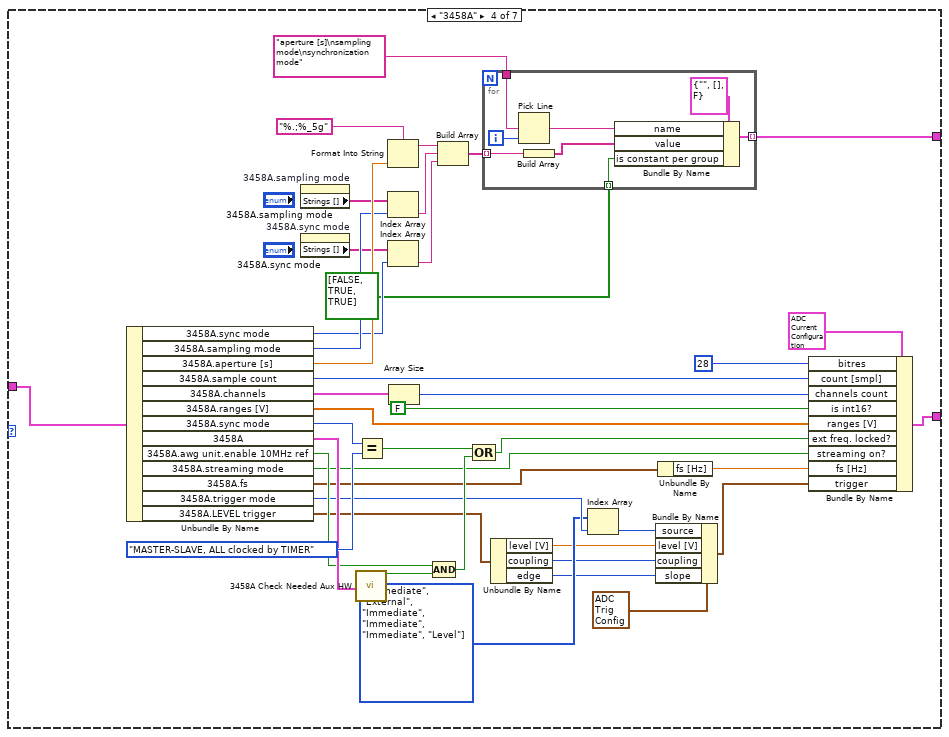
[diagram p4: hidden frame]
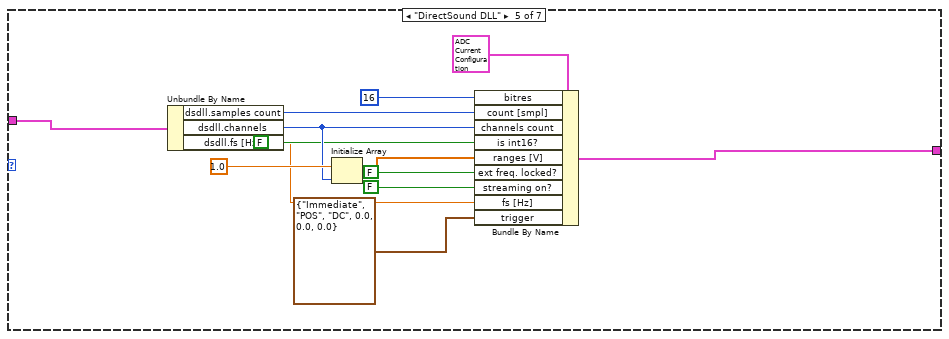
[diagram p5: hidden frame]
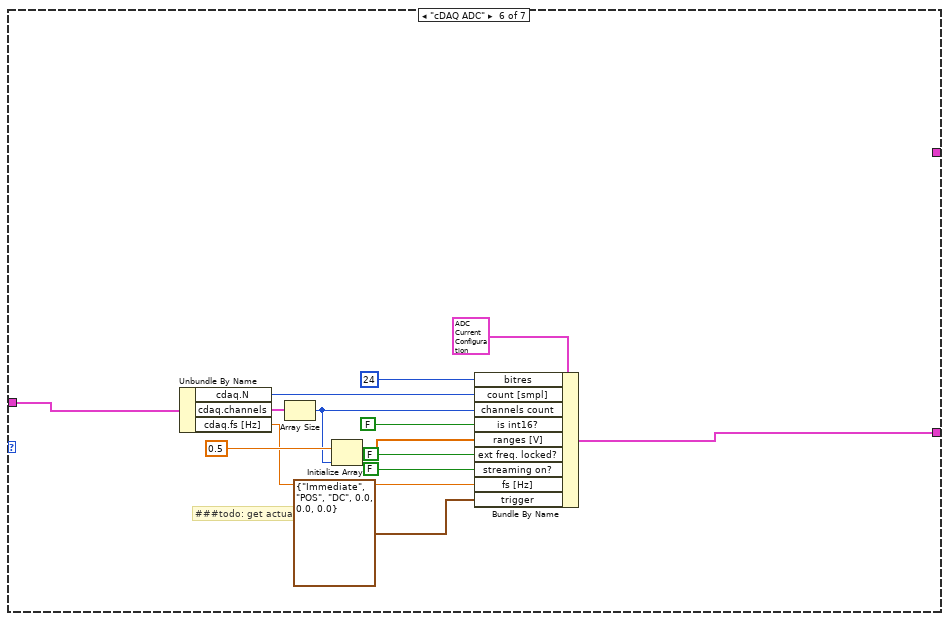
[diagram p6: hidden frame]
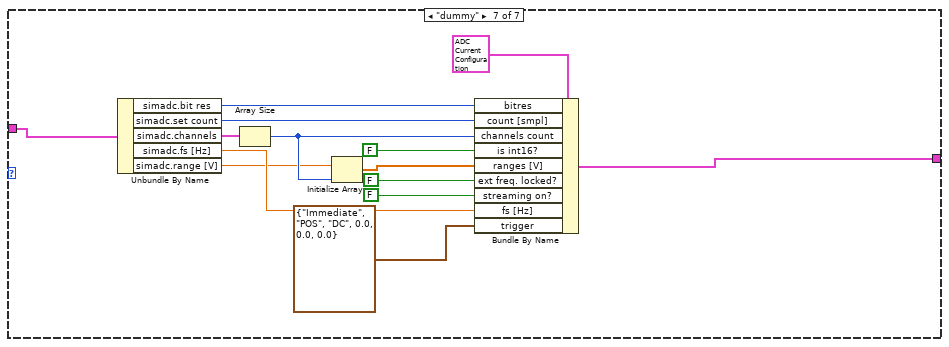
[diagram p7: hidden frame]
diagram:
  n1 = Unbundle By Name("adc session in") -> ("type"=w5:T60)
  n2 = case shown="\"CMI ADS127L21\"" w5 {
    tunnel: "adc session in" -> [w34 w61 w123 w185 w206 w220 w234]
    tunnel: [w8 w63 w108 w172 _ _ _] -> w2
    tunnel: [w23 w70 w119 w158 w197 w211 w227] -> w1
    frame "niScope", Default {
      n3 = Unbundle By Name(w34) -> ("niScope.bitres [bit]"=w7:i32, "niScope.channel cfg"=w14:T16[], "niScope.samples count"=w30:i64, "niScope.channels"=w29:i32, "niScope.sample width [B]"=w33:i32, "niScope.ranges [V]"=w27:dbl[], "niScope.ext. clock [Hz]"=w26:dbl, "niScope.use streaming"=w24:bool, "niScope.fs [Hz]"=w22:dbl, "niScope.trigger setup"=w21:T19)
      n4 = Unbundle By Name(w21) -> ("coupling"=w19:T20, "level [V]"=w18:dbl, "slope"=w17:T21, "mode"=w16:enum16{"Immediate", "External", "Level"})
      n5 = for {
        tunnel: w14 -> [w51] mode=indexing
        tunnel: [w48] -> w12 mode=indexing
        tunnel: [w45] -> w11 mode=indexing
        tunnel: [w42] -> w10 mode=indexing
        n6 = Unbundle By Name(w51) -> ("Mode"=w50:T5, "Input Z"=w46:T4, "Coupling"=w43:T3)
        n7 = property on="Coupling" class="Enum (strict)"() -> ("Strings []"=w44:string[])  [unwired: 2 in, 2 out]
        n8 = property on="Input Z" class="Enum (strict)"() -> ("Strings []"=w47:string[])  [unwired: 2 in, 2 out]
        n9 = property on="Mode" class="Enum (strict)"() -> ("Strings []"=w49:string[])  [unwired: 2 in, 2 out]
        n10 = Index Array(array=w49, index=w50) -> (element=w48:string)
        n11 = Index Array(array=w47, index=w46) -> (element=w45:string)
        n12 = Index Array(array=w44, index=w43) -> (element=w42:string)
      }
      n13 = Greater Than 0?(x=w26) -> (x > 0?=w25:bool)
      n14 = Equal?(x=w33, y=2) -> (x = y?=w28:bool)
      n15 = Bundle By Name(cluster=T7 {"source"=enum."Immediate", "slope"=enum."POS", "coupling"=enum."DC", "level [V]"=0.0, "hysteresis [V]"=0.0, "pre-trigger [%]"=0.0} ("trigger"), "coupling"=w19, "level [V]"=w18, "slope"=w17, "source"=w16) -> (w15:T7)
      n16 = Bundle By Name(cluster=T6 {"count [smpl]"=0, "channels count"=0, "fs [Hz]"=0.0, "ranges [V]"=[], "trigger"={"source"=enum."Immediate", "slope"=enum."POS", "coupling"=enum."DC", "level [V]"=0.0, "hysteresis [V]"=0.0, "pre-trigger [%]"=0.0}, "ext freq. locked?"=FALSE, "streaming on?"=FALSE, "is int16?"=FALSE, "bitres"=0} ("common attributes"), "bitres"=w7, "count [smpl]"=w30, "channels count"=w29, "is int16?"=w28, "ranges [V]"=w27, "ext freq. locked?"=w25, "streaming on?"=w24, "fs [Hz]"=w22, "trigger"=w15) -> (w23:T6)
      n17 = Build Array(w12, w11, w10) -> (w9:string[][])
      n18 = for {
        tunnel: "channel input mode\nchannel input Z\nchannel coupling" -> [w40]
        tunnel: [w37] -> w8 mode=indexing
        tunnel: w9 -> [w36] mode=indexing
        tunnel: bool[] [TRUE, TRUE, TRUE] -> [w35] mode=indexing
        i -> [w39]
        n19 = Pick Line(multi-line string=w40, line index=w39) -> (output string=w38:string)  [unwired: 1 in]
        n20 = Bundle By Name(cluster=T11 {"name"="", "value"=[], "is constant per group"=FALSE} ("adc attribute"), "name"=w38, "value"=w36, "is constant per group"=w35) -> (w37:T11)
      }
    }
    frame "CMI ADS127L21" {
      n21 = Unbundle By Name(w61) -> ("ADS127L21"=w60:T85)
      n22 = Unbundle By Name(w60) -> ("channels"=w68:T86[], "record size"=w71:i32, "channels"=w56:T86[], "ext refclk?"=w54:bool, "fs [Hz]"=w69:dbl)
      n23 = for {
        tunnel: w56 -> [w76] mode=indexing
        tunnel: [w73] -> w55 mode=indexing
        n24 = Unbundle By Name(w76) -> ("Range"=w75:T87)
        n25 = Index Array(array=dbl[] [1.65, 2.0], index=w75) -> (element=w73:dbl)
      }
      n26 = for {
        tunnel: w68 -> [w90] mode=indexing
        tunnel: [w88] -> w66 mode=indexing
        tunnel: [w86] -> w65 mode=indexing
        n27 = Unbundle By Name(w90) -> ("Mode"=w89:T2, "Impedance"=w87:T1)
        n28 = property on="ads127 Impedance" class="Enum (strict)"() -> ("Strings []"=w84:string[])  [unwired: 2 in, 2 out]
        n29 = property on="ads127 Mode" class="Enum (strict)"() -> ("Strings []"=w85:string[])  [unwired: 2 in, 2 out]
        n30 = Index Array(array=w85, index=w89) -> (element=w88:string)
        n31 = Index Array(array=w84, index=w87) -> (element=w86:string)
      }
      n32 = Array Size(array=w56) -> (size(s)=w58:i32)
      n33 = Bundle By Name(cluster=T6 {"count [smpl]"=0, "channels count"=0, "fs [Hz]"=0.0, "ranges [V]"=[], "trigger"={"source"=enum."Immediate", "slope"=enum."POS", "coupling"=enum."DC", "level [V]"=0.0, "hysteresis [V]"=0.0, "pre-trigger [%]"=0.0}, "ext freq. locked?"=FALSE, "streaming on?"=FALSE, "is int16?"=FALSE, "bitres"=0} ("common attributes"), "bitres"=24, "count [smpl]"=w71, "channels count"=w58, "is int16?"=FALSE, "ranges [V]"=w55, "ext freq. locked?"=w54, "streaming on?"=TRUE, "fs [Hz]"=w69, "trigger"=T7 {"source"=enum."Immediate", "slope"=enum."POS", "coupling"=enum."DC", "level [V]"=0.0, "hysteresis [V]"=0.0, "pre-trigger [%]"=0.0}) -> (w70:T6)
      n34 = Build Array(w66, w65) -> (w64:string[][])
      n35 = for {
        tunnel: "channel input mode\nchannel input Z" -> [w82]
        tunnel: [w79] -> w63 mode=indexing
        tunnel: w64 -> [w78] mode=indexing
        tunnel: bool[] [TRUE, TRUE] -> [w77] mode=indexing
        i -> [w81]
        n36 = Pick Line(multi-line string=w82, line index=w81) -> (output string=w80:string)  [unwired: 1 in]
        n37 = Bundle By Name(cluster=T11 {"name"="", "value"=[], "is constant per group"=FALSE} ("adc attribute"), "name"=w80, "value"=w78, "is constant per group"=w77) -> (w79:T11)
      }
    }
    frame "Keysight DSO" {
      w93 = T8[] [enum."Immediate", enum."Level", enum."External"] items=["Immediate", "External", "Level"]
      w97 = T9[] [enum."NEG", enum."POS"] items=["POS", "NEG"]
      # "###todo: auto should be read from instr? Default: 8b"
      n38 = Unbundle By Name(w123) -> ("keysight dso.bw limit [Hz]"=w91:dbl, "keysight dso.resolution"=w104:T78, "keysight dso.channels"=w103:T77[], "keysight dso.N"=w121:i64, "keysight dso.ranges [V]"=w120:dbl[], "keysight dso.fs [Hz]"=w118:dbl, "keysight dso.trigger config"=w117:T79)
      n39 = Unbundle By Name(w117) -> ("level [V]"=w115:dbl, "trigger slope"=w96:enum16{"Negative", "Positive", "Either"}, "trigger source"=w94:T80)
      n40 = Array Size(array=w103) -> (size(s)=w102:i32)
      n41 = for {
        tunnel: w103 -> [w143] mode=indexing
        tunnel: [w139] -> w112 mode=indexing
        tunnel: [w137] -> w111 mode=indexing
        tunnel: [w141] -> w110 mode=indexing
        tunnel: w91 -> [w131]
        n42 = Unbundle By Name(w143) -> ("bw limit enab"=w138:bool, "Offset [V]"=w136:dbl, "Coupling"=w142:enum16{"DC", "DC50", "AC", "LFR1"})
        n43 = property on="Coupling 2" class="Enum (strict)"() -> ("Strings []"=w140:string[])  [unwired: 2 in, 2 out]
        n44 = Format Into String(format string="%.;%_4g", w131) -> (resulting string=w132:string)  [unwired: 2 in, 1 out]
        n45 = Format Into String(format string="%.;%_4g", w136) -> (resulting string=w137:string)  [unwired: 2 in, 1 out]
        n46 = Index Array(array=w140, index=w142) -> (element=w141:string)
        n47 = Select(t=w132, s=w138, f="inf" ("format string")) -> (s? t:f=w139:string)
      }
      n48 = Index Array(array=w97, index=w96) -> (element=w95:T9)
      n49 = Index Array(array=w93, index=w94) -> (element=w92:T8)
      n50 = Bundle By Name(cluster=T7 {"source"=enum."Immediate", "slope"=enum."POS", "coupling"=enum."DC", "level [V]"=0.0, "hysteresis [V]"=0.0, "pre-trigger [%]"=0.0} ("trigger"), "coupling"=ADC_Trig_Coupling."DC", "level [V]"=w115, "slope"=w95, "source"=w92) -> (w114:T7)
      n51 = Index Array(array=i32[] [8, 9, 10, 11, 12], index=w104) -> (element=w105:i32)
      n52 = Bundle By Name(cluster=T6 {"count [smpl]"=0, "channels count"=0, "fs [Hz]"=0.0, "ranges [V]"=[], "trigger"={"source"=enum."Immediate", "slope"=enum."POS", "coupling"=enum."DC", "level [V]"=0.0, "hysteresis [V]"=0.0, "pre-trigger [%]"=0.0}, "ext freq. locked?"=FALSE, "streaming on?"=FALSE, "is int16?"=FALSE, "bitres"=0} ("common attributes"), "bitres"=w105, "count [smpl]"=w121, "channels count"=w102, "is int16?"=TRUE, "ranges [V]"=w120, "ext freq. locked?"=FALSE, "streaming on?"=FALSE, "fs [Hz]"=w118, "trigger"=w114) -> (w119:T6)
      n53 = Build Array(w112, w111, w110) -> (w109:string[][])
      n54 = for {
        tunnel: "channel bandwidth limits [Hz]\nchannel offset [V]\nchannel coupling mode " -> [w129]
        tunnel: [w126] -> w108 mode=indexing
        tunnel: w109 -> [w125] mode=indexing
        tunnel: bool[] [TRUE, TRUE, TRUE] -> [w124] mode=indexing
        i -> [w128]
        n55 = Pick Line(multi-line string=w129, line index=w128) -> (output string=w127:string)  [unwired: 1 in]
        n56 = Bundle By Name(cluster=T11 {"name"="", "value"=[], "is constant per group"=FALSE} ("adc attribute"), "name"=w127, "value"=w125, "is constant per group"=w124) -> (w126:T11)
      }
    }
    frame "3458A" {
      w154 = T8[] [enum."Immediate", enum."External", enum."Immediate", enum."Immediate", enum."Immediate", enum."Level"] items=["Immediate", "External", "Level"]
      n57 = Unbundle By Name(w185) -> ("3458A.sync mode"=w178:T12, "3458A.sampling mode"=w180:T13, "3458A.aperture [s]"=w182:dbl, "3458A.sample count"=w170:i32, "3458A.channels"=w184:T24[], "3458A.ranges [V]"=w168:dbl[], "3458A.sync mode"=w167:T12, "3458A"=w163:T23, "3458A.awg unit.enable 10MHz ref"=w162:bool, "3458A.streaming mode"=w159:bool, "3458A.fs"=w145:T53, "3458A.trigger mode"=w155:T47, "3458A.LEVEL trigger"=w152:T46)
      n58 = property on="3458A.sampling mode" class="Enum (strict)"() -> ("Strings []"=w181:string[])  [unwired: 2 in, 2 out]
      n59 = property on="3458A.sync mode" class="Enum (strict)"() -> ("Strings []"=w179:string[])  [unwired: 2 in, 2 out]
      n60 = call "3458A Check Needed Aux HW.vi"("digitizer session"=w163) -> ("uses AWG clocking?"=w161:bool)  [unwired: 13 in, 5 out]
      n61 = Equal?(x=w167, y=3458A_Sync_Mode."MASTER-SLAVE, ALL clocked by TIMER") -> (x = y?=w165:bool)
      n62 = Format Into String(format string="%.;%_5g", w182) -> (resulting string=w176:string)  [unwired: 2 in, 1 out]
      n63 = Index Array(array=w181, index=w180) -> (element=w175:string)
      n64 = Index Array(array=w179, index=w178) -> (element=w174:string)
      n65 = Array Size(array=w184) -> (size(s)=w148:i32)
      n66 = Compound Arithmetic op=AND(w162, w161) -> (w160:bool)
      n67 = Build Array(w176, w175, w174) -> (w173:string[])
      n68 = Compound Arithmetic op=OR(w165, w160) -> (w164:bool)
      n69 = for {
        tunnel: "aperture [s]\nsampling mode\nsynchronization mode" -> [w192]
        tunnel: [w189] -> w172 mode=indexing
        tunnel: w173 -> [w188] mode=indexing
        tunnel: bool[] [FALSE, TRUE, TRUE] -> [w186] mode=indexing
        i -> [w191]
        n70 = Pick Line(multi-line string=w192, line index=w191) -> (output string=w190:string)  [unwired: 1 in]
        n71 = Build Array(w188) -> (w187:string[])
        n72 = Bundle By Name(cluster=T11 {"name"="", "value"=[], "is constant per group"=FALSE} ("adc attribute"), "name"=w190, "value"=w187, "is constant per group"=w186) -> (w189:T11)
      }
      n73 = Unbundle By Name(w152) -> ("level [V]"=w151:dbl, "coupling"=w150:enum16{"DC", "AC"}, "edge"=w149:enum16{"POS", "NEG"})
      n74 = Index Array(array=w154, index=w155) -> (element=w153:T8)
      n75 = Bundle By Name(cluster=T7 {"source"=enum."Immediate", "slope"=enum."POS", "coupling"=enum."DC", "level [V]"=0.0, "hysteresis [V]"=0.0, "pre-trigger [%]"=0.0} ("trigger"), "source"=w153, "level [V]"=w151, "coupling"=w150, "slope"=w149) -> (w156:T7)
      n76 = Unbundle By Name(w145) -> ("fs [Hz]"=w144:dbl)
      n77 = Bundle By Name(cluster=T6 {"count [smpl]"=0, "channels count"=0, "fs [Hz]"=0.0, "ranges [V]"=[], "trigger"={"source"=enum."Immediate", "slope"=enum."POS", "coupling"=enum."DC", "level [V]"=0.0, "hysteresis [V]"=0.0, "pre-trigger [%]"=0.0}, "ext freq. locked?"=FALSE, "streaming on?"=FALSE, "is int16?"=FALSE, "bitres"=0} ("common attributes"), "bitres"=28, "count [smpl]"=w170, "channels count"=w148, "is int16?"=FALSE, "ranges [V]"=w168, "ext freq. locked?"=w164, "streaming on?"=w159, "fs [Hz]"=w144, "trigger"=w156) -> (w158:T6)
    }
    frame "DirectSound DLL" {
      n78 = Unbundle By Name(w206) -> ("dsdll.samples count"=w203:i32, "dsdll.channels"=w202:i32, "dsdll.fs [Hz]"=w196:dbl)
      n79 = Initialize Array(1.0 ("element"), w202) -> (w200:dbl[])
      n80 = Bundle By Name(cluster=T6 {"count [smpl]"=0, "channels count"=0, "fs [Hz]"=0.0, "ranges [V]"=[], "trigger"={"source"=enum."Immediate", "slope"=enum."POS", "coupling"=enum."DC", "level [V]"=0.0, "hysteresis [V]"=0.0, "pre-trigger [%]"=0.0}, "ext freq. locked?"=FALSE, "streaming on?"=FALSE, "is int16?"=FALSE, "bitres"=0} ("common attributes"), "bitres"=16, "count [smpl]"=w203, "channels count"=w202, "is int16?"=FALSE, "ranges [V]"=w200, "ext freq. locked?"=FALSE, "streaming on?"=FALSE, "fs [Hz]"=w196, "trigger"=T7 {"source"=enum."Immediate", "slope"=enum."POS", "coupling"=enum."DC", "level [V]"=0.0, "hysteresis [V]"=0.0, "pre-trigger [%]"=0.0}) -> (w197:T6)
    }
    frame "cDAQ ADC" {
      # "###todo: get actual range"
      n81 = Unbundle By Name(w220) -> ("cdaq.N"=w217:i32, "cdaq.channels"=w216:T83[], "cdaq.fs [Hz]"=w210:dbl)
      n82 = Array Size(array=w216) -> (size(s)=w207:i32)
      n83 = Initialize Array(0.5 ("element"), w207) -> (w214:dbl[])
      n84 = Bundle By Name(cluster=T6 {"count [smpl]"=0, "channels count"=0, "fs [Hz]"=0.0, "ranges [V]"=[], "trigger"={"source"=enum."Immediate", "slope"=enum."POS", "coupling"=enum."DC", "level [V]"=0.0, "hysteresis [V]"=0.0, "pre-trigger [%]"=0.0}, "ext freq. locked?"=FALSE, "streaming on?"=FALSE, "is int16?"=FALSE, "bitres"=0} ("common attributes"), "bitres"=24, "count [smpl]"=w217, "channels count"=w207, "is int16?"=FALSE, "ranges [V]"=w214, "ext freq. locked?"=FALSE, "streaming on?"=FALSE, "fs [Hz]"=w210, "trigger"=T7 {"source"=enum."Immediate", "slope"=enum."POS", "coupling"=enum."DC", "level [V]"=0.0, "hysteresis [V]"=0.0, "pre-trigger [%]"=0.0}) -> (w211:T6)
    }
    frame "dummy" {
      n85 = Unbundle By Name(w234) -> ("simadc.bit res"=w221:i32, "simadc.set count"=w232:i64, "simadc.channels"=w224:T62[], "simadc.fs [Hz]"=w226:dbl, "simadc.range [V]"=w222:dbl)
      n86 = Array Size(array=w224) -> (size(s)=w223:i32)
      n87 = Initialize Array(w222, w223) -> (w230:dbl[])
      n88 = Bundle By Name(cluster=T6 {"count [smpl]"=0, "channels count"=0, "fs [Hz]"=0.0, "ranges [V]"=[], "trigger"={"source"=enum."Immediate", "slope"=enum."POS", "coupling"=enum."DC", "level [V]"=0.0, "hysteresis [V]"=0.0, "pre-trigger [%]"=0.0}, "ext freq. locked?"=FALSE, "streaming on?"=FALSE, "is int16?"=FALSE, "bitres"=0} ("common attributes"), "bitres"=w221, "count [smpl]"=w232, "channels count"=w223, "is int16?"=FALSE, "ranges [V]"=w230, "ext freq. locked?"=FALSE, "streaming on?"=FALSE, "fs [Hz]"=w226, "trigger"=T7 {"source"=enum."Immediate", "slope"=enum."POS", "coupling"=enum."DC", "level [V]"=0.0, "hysteresis [V]"=0.0, "pre-trigger [%]"=0.0}) -> (w227:T6)
    }
  }
  "device specific attributes" <- w2
  "common attributes" <- w1
  "error out" <- "error in"
  "adc session out" <- "adc session in"
